vi "Bit_to_byte.vi"(8 "Error In":errorcluster, 10 "Array of bit":u8[](array[numeric])=[0, 1, 1, 0, 0, 0, 0, 0]) -> (0 "Error Out":errorcluster, 1 "BYTE":string, 2 "Array of byte":u8[](array[numeric]))   [LabVIEW 2019]
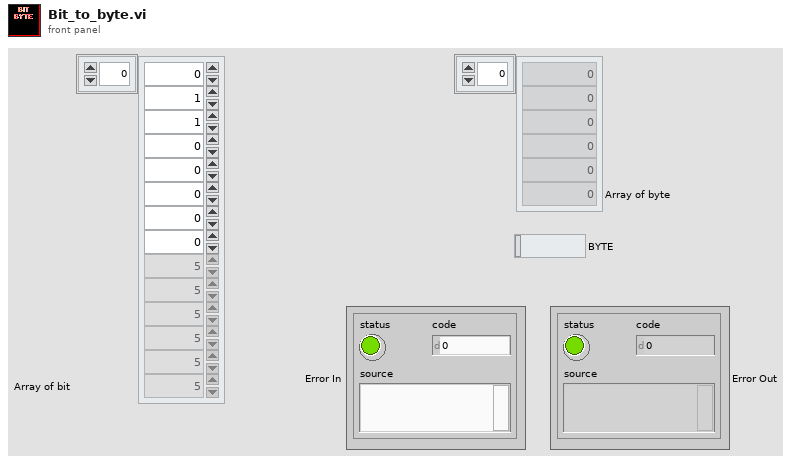
[diagram p1: front panel]
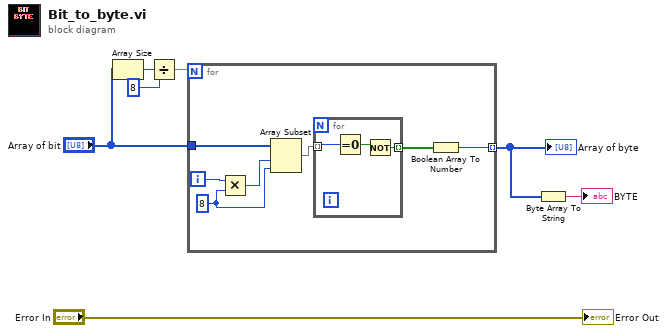
[diagram p0: block diagram]
diagram:
  n1 = Array Size(array="Array of bit") -> (size(s)=w6:i32)
  n2 = Divide(x=w6, y=8) -> (x/y=w5:dbl)
  n3 = for {
    N: w5 -> [_]
    tunnel: "Array of bit" -> [w10]
    tunnel: [w13] -> w3 mode=indexing
    i -> [w12]
    w8 = u8 8 ("y")
    n4 = Multiply(x=w12, y=w8) -> (x*y=w9:i32)
    n5 = Array Subset(array=w10, index=w9, length=w8) -> (w11:u8[])
    n6 = for {
      tunnel: [w16] -> w14 mode=indexing
      tunnel: w11 -> [w15] mode=indexing
      n7 = Equal To 0?(x=w15) -> (x = 0?=w17:bool)
      n8 = Not(x=w17) -> (.not. x?=w16:bool)
    }
    n9 = Boolean Array To Number(Boolean array=w14) -> (number=w13:u32)
  }
  "Array of byte" <- w3
  n10 = Byte Array To String(unsigned byte array=w3) -> (string=→"BYTE":string)
  "Error Out" <- "Error In"
